vi "Test Log.vi"(7 "Name":string="Test Log", 11 "Message":string) -> (3 "BT.lvlib:abs_Node.lvclass":refnum<class "abs_Node.lvclass">)   [LabVIEW 2021]
uses:
  abs_Node/abs_Node.lvclass
  Test Log.lvclass
  C:/Users/Tim/Documents/LabVIEW/2021/Behaviour Tree/Source/abs_Log/abs_Log.lvclass
  C:/Users/Tim/Documents/LabVIEW/2021/Behaviour Tree/Source/abs_Node/abs_Node.lvclass
  abs_Log/abs_Log.lvclass/abs_Log.ctl
  abs_Node/abs_Node.lvclass/abs_Node.ctl
  abs_Log/Properties/Write Message.vi
  abs_Node/Properties/Write Name.vi
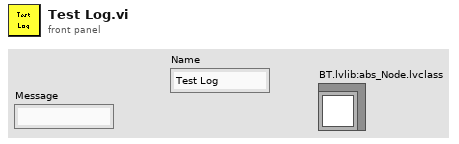
[diagram p1: front panel]
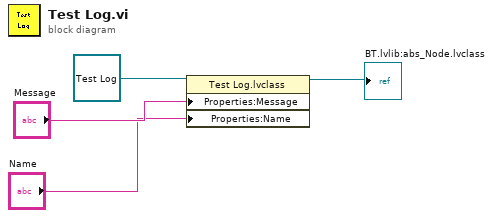
[diagram p0: block diagram]
diagram:
  n1 = property class="Test Log.lvclass"(reference=refnum<class "Test Log.lvclass"> refnum ("Test Log.lvclass"), "Properties:Message"="Message", "Properties:Name"="Name") -> (reference out=→"BT.lvlib:abs_Node.lvclass":refnum<class "Test Log.lvclass">)  [unwired: 1 in, 1 out]
